vi "Insert book exchange into jos_menu.vi"(1 "id of content article":string, 3 "title":string) -> ()   [LabVIEW 2010]
doc: "This example opens a connection to a database specified by the Connection string (replace the DNS name with your database) inserts a new row into the table \"myOtherTable\" (replace the SQL string with your own SQL query)."
panel:
  out "concatenated string":string
  out "error out":errorcluster
  in  "Command Text":string="INSERT INTO jos_menu\n (id, menutype, name, alias, link to article, type, published, parent, componentid, sublevel, browserNav, access, utaccess, params, lft, rgt, home)\nVALUES ('id', 'unpublished', 'name', 'alias', 'index.php?option=com_content&view=article&id=117', 'component', '1', '0', '20', '0', '0', '0', '0', 'show_noauth=\nshow_title=\nlink_titles=\nshow_intro=\nshow_section=\nlink_section=\nshow_category=\nlink_category=\nshow_author=\nshow_create_date=\nshow_modify_date=\nshow_item_navigation=\nshow_readmore=\nshow_vote=\nshow_icons=\nshow_pdf_icon=\nshow_print_icon=\nshow_email_icon=\nshow_hits=\nfeed_summary=\npage_title=\nshow_page_title=1\npageclass_sfx=\nmenu_image=-1\nsecure=0\n', '0', '0', '0');"
  in  "ConnectionString":string="DSN=stusbooks;"
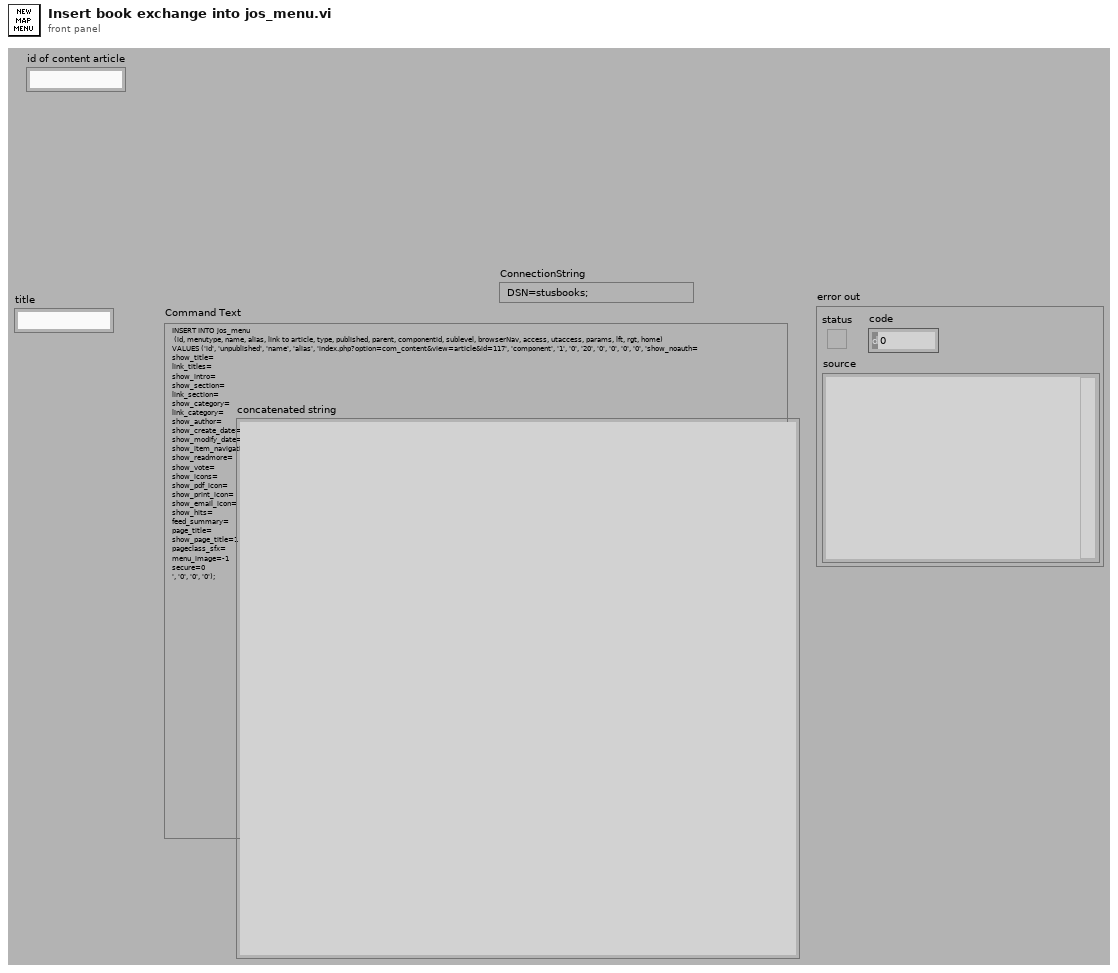
[diagram p1: front panel]
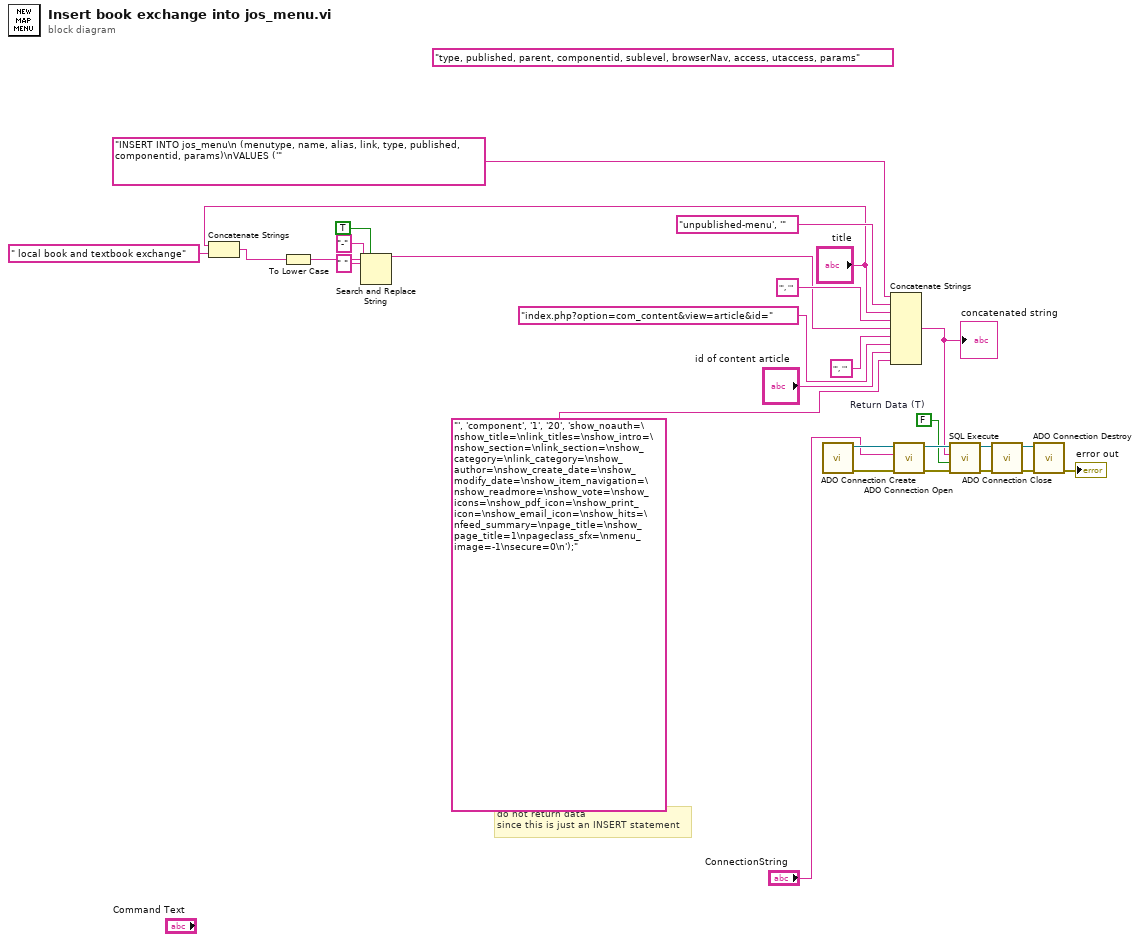
[diagram p0: block diagram]
diagram:
  (unwired) "type, published, parent, componentid, sublevel, browserNav, access, utaccess, params"
  w17 = FALSE  # Return Data (T)
  # "do not return data\nsince this is just an INSERT statement"
  n1 = Concatenate Strings("title", " local book and textbook exchange" ("string")) -> (w2:string)
  n2 = To Lower Case(string=w2) -> (all lower case string=w8:string)
  n3 = Search and Replace String(replace all?=TRUE ("replace all? (F)"), input string=w8, search string=" ", replace string="-" ("replace string (\"\")")) -> (result string=w1:string)  [unwired: 4 in, 3 out]
  n4 = call "ADO Connection Create.vi"() -> ("error out"=w26:errorcluster, "ADODB._Connection Out"=w27:refnum<k7>)  [unwired: 10 in]
  n5 = Concatenate Strings("INSERT INTO jos_menu\n (menutype, name, alias, link, type, published, componentid, params)\nVALUES ('", "unpublished-menu', '" ("string"), "title", "', '" ("string"), w1, "', '" ("string"), "index.php?option=com_content&view=article&id=", "id of content article", "', 'component', '1', '20', 'show_noauth=\nshow_title=\nlink_titles=\nshow_intro=\nshow_section=\nlink_section=\nshow_category=\nlink_category=\nshow_author=\nshow_create_date=\nshow_modify_date=\nshow_item_navigation=\nshow_readmore=\nshow_vote=\nshow_icons=\nshow_pdf_icon=\nshow_print_icon=\nshow_email_icon=\nshow_hits=\nfeed_summary=\npage_title=\nshow_page_title=1\npageclass_sfx=\nmenu_image=-1\nsecure=0\n');" ("string")) -> (w11:string)
  "concatenated string" <- w11
  n6 = call "ADO Connection Open.vi"("error in (no error)"=w26, "ConnectionString"="ConnectionString", "ADODB._Connection In"=w27) -> ("error out"=w23:errorcluster, "ADODB._Connection Out"=w24:refnum<k7>)  [unwired: 7 in]
  n7 = call "SQL Execute.vi"("error in (no error)"=w23, "Return Data (T)"=w17, "Command Text"=w11, "ADODB._Connection In"=w24) -> ("error out"=w22:errorcluster, "ADODB._Connection Out"=w21:refnum<k7>)  [unwired: 4 in, 2 out]
  n8 = call "ADO Connection Close.vi"("error in (no error)"=w22, "ADODB._Connection In"=w21) -> ("error out"=w20:errorcluster, "ADODB._Connection Out"=w19:refnum<k7>)  [unwired: 8 in]
  n9 = call "ADO Connection Destroy.vi"("error in (no error)"=w20, "ADODB._Connection In"=w19) -> ("error out"=→"error out":errorcluster)  [unwired: 9 in]
